vi "Is OceanOptics installed.vi"(8 "Error In":errorcluster) -> (0 "Error Out":errorcluster, 3 "file or folder exists?":bool)   [LabVIEW 2019]
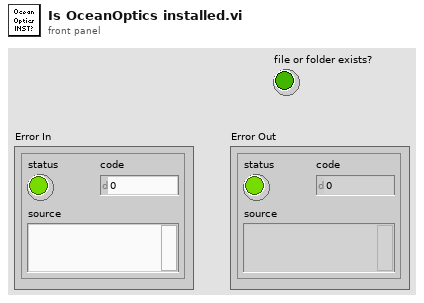
[diagram p1: front panel]
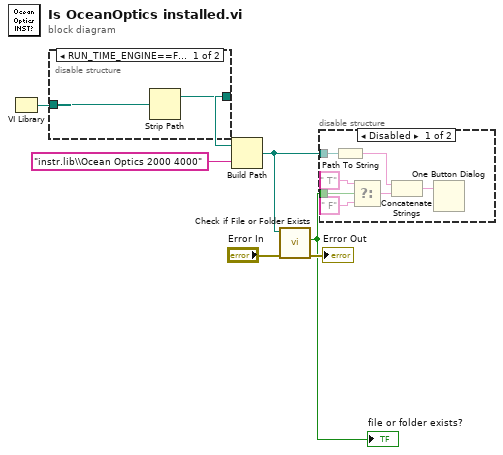
[diagram p0: block diagram]
diagram:
  n1 = VI Library() -> (path=w4:path)
  n2 = disable-structure shown="RUN_TIME_ENGINE==False, Default" {
    disable-tunnel: w4 -> [w9 w10]
    disable-tunnel: [w8 w10] -> w3
    frame condition #0 (active) {
      n3 = Strip Path(path=w9) -> (stripped path=w8:path)  [unwired: 1 out]
    }
    frame condition #1 {
    }
  }
  n4 = Build Path(base path=w3, name or relative path="instr.lib\\Ocean Optics 2000 4000") -> (appended path=w2:path)
  n5 = call <vilib>:"Check if File or Folder Exists.vi"("error in (no error)"="Error In", "path"=w2) -> ("error out"=→"Error Out":errorcluster, "file or folder exists?"=w1:bool)  [unwired: 7 in, 1 out]
  "file or folder exists?" <- w1
  n6 = disable-structure shown="Disabled" {
    disable-tunnel: w2 -> [w17 _]
    disable-tunnel: w1 -> [w14 _]
    frame Disabled {
      n7 = Path To String(path=w17) -> (string=w16:string)
      n8 = Select(t=" T" ("concatenated string"), s=w14, f=" F" ("concatenated string")) -> (s? t:f=w11:string)
      n9 = Concatenate Strings(w16, w11) -> (w15:string)
      n10 = One Button Dialog(message=w15) -> ()  [unwired: 1 in, 1 out]
    }
    frame Enabled {
    }
  }
